vi "acquireSinglePoint.vi"(2 "待读取长度":i32, 3 "量程":i32, 4 "设备输入":i32) -> (0 "ch1":dbl[](array[numeric]), 1 "ch0":dbl[](array[numeric]))   [LabVIEW 2018]
uses:
  PCI8552B_32.dll
panel:
  out "待读取数据长度":i32
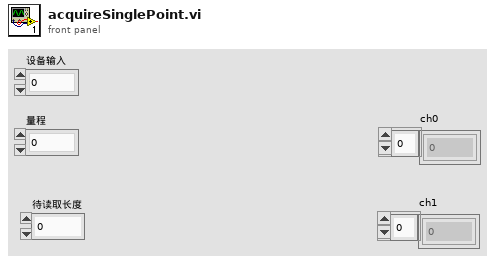
[diagram p1: front panel]
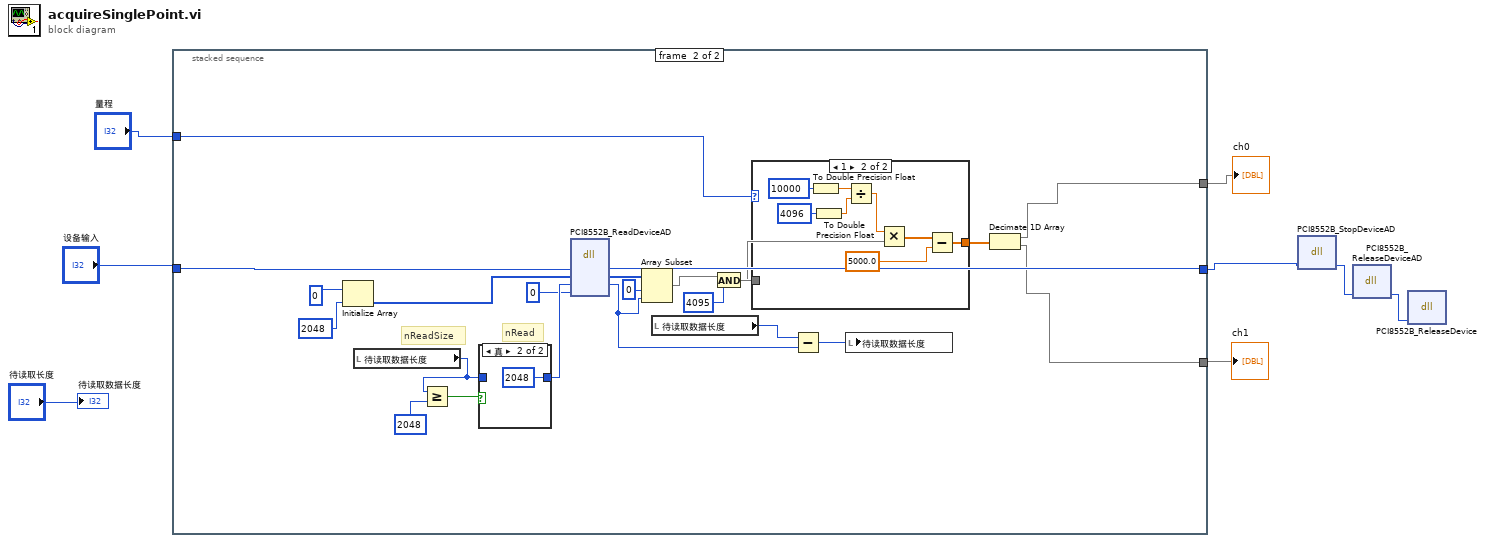
[diagram p0: block diagram]
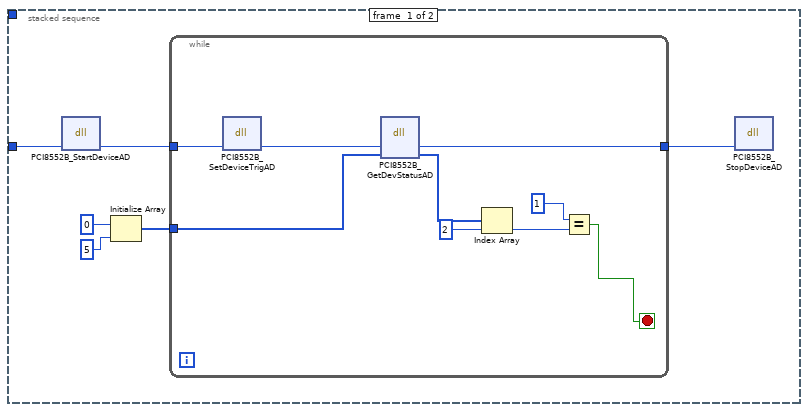
[diagram p2: hidden frame]
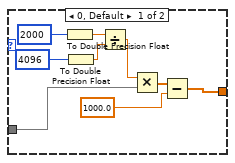
[diagram p3: hidden frame]
diagram:
  n1 = stacked-sequence {
    tunnel: "设备输入" -> [w10 w41]
    tunnel: [_ w45] -> w2
    tunnel: "量程" -> [_ w40]
    tunnel: [_ w39] -> w5
    tunnel: [_ w38] -> w4
    frame #0 {
      n2 = dll-call lib="PTH2pabs E\nPersonal File研究生学习202002-202007研一下学期work2020mmw_controllerPCI8552B_32.DLL" fn="PCI8552B_StartDeviceAD" label="StartDeviceAD"("hDevice"=w10) -> ("hDevice"=w9:i32)  [unwired: 4 in, 2 out]
      n3 = Initialize Array(0, 5) -> (w14:i32[])
      n4 = while {
        tunnel: w9 -> [w18]
        tunnel: w14 -> [w23]
        tunnel: [w16] -> w11
        stop <- w15 stop-if-true
        n5 = dll-call lib="PTH2pabs E\nPersonal File研究生学习202002-202007研一下学期work2020mmw_controllerPCI8552B_32.DLL" fn="PCI8552B_SetDeviceTrigAD" label="SetDeviceTrigAD"("hDevice"=w18) -> ("hDevice"=w17:i32)  [unwired: 4 in, 2 out]
        n6 = dll-call lib="PTH2pabs E\nPersonal File研究生学习202002-202007研一下学期work2020mmw_controllerPCI8552B_32.DLL" fn="PCI8552B_GetDevStatusAD" label="GetDevStatusAD"("hDevice"=w17, "ADStatus"=w23) -> ("hDevice"=w16:i32, "ADStatus"=w19:i32[])  [unwired: 4 in, 2 out]
        n7 = Index Array(array=w19, index=2) -> (element=w21:i32)
        n8 = Equal?(x=1, y=w21) -> (x = y?=w15:bool)
      }
      n9 = dll-call lib="PTH2pabs E\nPersonal File研究生学习202002-202007研一下学期work2020mmw_controllerPCI8552B_32.DLL" fn="PCI8552B_StopDeviceAD" label="StopDeviceAD"("hDevice"=w11) -> ()  [unwired: 5 in, 2 out]
    }
    frame #1 {
      # "nReadSize"
      # "nRead"
      n10 = Initialize Array(u16 0 ("y"), 2048 ("y")) -> (w42:u16[])
      n11 = local read "待读取数据长度"() -> (w35:i32)
      n12 = Greater Or Equal?(x=w35, y=2048 ("millisecond multiple")) -> (x >= y?=w36:bool)
      n13 = case shown="真" w36 {
        tunnel: [w64 2048 ("millisecond multiple")] -> w32
        tunnel: w35 -> [w64 _]
        frame False {
        }
        frame True {
        }
      }
      n14 = dll-call lib="PTH2pabs E\nPersonal File研究生学习202002-202007研一下学期work2020mmw_controllerPCI8552B_32.DLL" fn="PCI8552B_ReadDeviceAD" label="ReadDeviceAD"("hDevice"=w41, "pADBuffer"=w42, "nReadSizeWords"=w32, "nRetSizeWords"=0) -> ("hDevice"=w45:i32, "pADBuffer"=w27:u16[], "nReadSizeWords"=w24:u32)  [unwired: 5 in, 2 out]
      n15 = Array Subset(array=w27, index=0 ("索引"), length=w24) -> (w26:u16[])
      n16 = local read "待读取数据长度"() -> (w34:i32)
      n17 = And(x=w26, y=u16 4095) -> (x .and. y?=w30:u16[])
      n18 = case shown="1" w40 {
        tunnel: w30 -> [w53 w58]
        tunnel: [w46 w57] -> w29
        frame 0, Default {
          n19 = To Double Precision Float(number=2000 ("x")) -> (double precision float=w49:dbl)
          n20 = To Double Precision Float(number=4096) -> (double precision float=w48:dbl)
          n21 = Divide(x=w49, y=w48) -> (x/y=w54:dbl)
          n22 = Multiply(x=w54, y=w53) -> (x*y=w52:dbl[])
          n23 = Subtract(x=w52, y=1000.0) -> (x-y=w46:dbl[])
        }
        frame 1 {
          n24 = To Double Precision Float(number=10000 ("x")) -> (double precision float=w56:dbl)
          n25 = To Double Precision Float(number=4096) -> (double precision float=w60:dbl)
          n26 = Divide(x=w56, y=w60) -> (x/y=w63:dbl)
          n27 = Multiply(x=w63, y=w58) -> (x*y=w62:dbl[])
          n28 = Subtract(x=w62, y=5000.0) -> (x-y=w57:dbl[])
        }
      }
      n29 = Subtract(x=w34, y=w24) -> (x-y=w33:u32)
      n30 = local write "待读取数据长度"(w33) -> ()
      n31 = Decimate 1D Array(w29) -> (w39:dbl[], w38:dbl[])
    }
  }
  "ch0" <- w5
  "ch1" <- w4
  n32 = dll-call lib="PTH2pabs E\nPersonal File研究生学习202002-202007研一下学期work2020mmw_controllerPCI8552B_32.DLL" fn="PCI8552B_StopDeviceAD" label="StopDeviceAD"("hDevice"=w2) -> ("hDevice"=w3:i32)  [unwired: 4 in, 2 out]
  n33 = dll-call lib="PTH2pabs E\nPersonal File研究生学习202002-202007研一下学期work2020mmw_controllerPCI8552B_32.DLL" fn="PCI8552B_ReleaseDeviceAD" label="ReleaseDeviceAD"("hDevice"=w3) -> ("hDevice"=w1:i32)  [unwired: 4 in, 2 out]
  n34 = dll-call lib="PTH2pabs E\nPersonal File研究生学习202002-202007研一下学期work2020mmw_controllerPCI8552B_32.DLL" fn="PCI8552B_ReleaseDevice" label="ReleaseDevice"("hDevice"=w1) -> ()  [unwired: 5 in, 2 out]
  "待读取数据长度" <- "待读取长度"
